vi "Update All Elec Grid Controls.vi"(8 "Error In":errorcluster, 9 "Bitmask":u64, 10 "Electrode Grid Objects (XS to LG)":refnum<class "ElectrodeGrid.lvclass">[](array[class]), 11 "Refs to Electrode Controls (XS to LG)":refnum<vi>[](array[refnum])) -> (0 "Error Out":errorcluster)   [LabVIEW 2017]
doc: "This VI updates an array of references to the XS, SM and LG electrode grid controls.\n\nParams: Array of refs to controls (ordered XS -> LG), array of electrode grid objects (ordered XS -> LG), bitmask to write, error in."
uses:
  Classes/ElectrodeGrid.lvclass
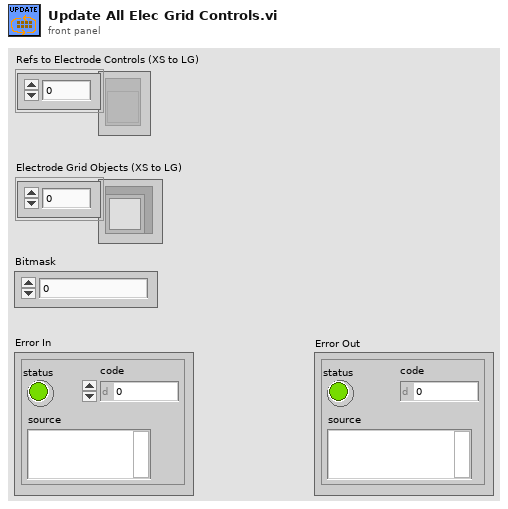
[diagram p1: front panel]
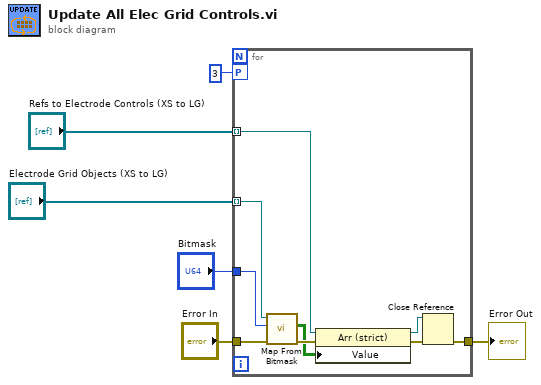
[diagram p0: block diagram]
diagram:
  n1 = for {
    tunnel: "Electrode Grid Objects (XS to LG)" -> [w15] mode=indexing
    workers-P: 3 -> [_]
    tunnel: "Refs to Electrode Controls (XS to LG)" -> [w11] mode=indexing
    tunnel: "Bitmask" -> [w14]
    tunnel: "Error In" -> [w13]
    tunnel: [w7] -> w1
    n2 = call "Map From Bitmask.vi"("error in (no error)"=w13, "Bitmask"=w14, "ElectrodeGrid in"=w15) -> ("error out"=w12:errorcluster, "Elec Grid Output"=w10:bool[][])  [unwired: 6 in, 1 out]
    n3 = property class="Arr (strict)"(reference=w11, error in=w12, "Value"=w10) -> (reference out=w8:refnum<vi>, error out=w9:errorcluster)
    n4 = Close Reference(reference=w8, error in (no error)=w9) -> (error out=w7:errorcluster)
  }
  "Error Out" <- w1
